vi "Read.vi"(8 "error in (no error)":errorcluster, 10 "maximum time (5s)":dbl[unit]=5000.0 caption="maximum time (5000 ms)", 11 "IVI_DMM in":refnum<class "IVI_DMM.lvclass">) -> (0 "error out":errorcluster, 2 "reading":dbl format="%^.2e", 3 "IVI_DMM out":refnum<class "IVI_DMM.lvclass">)   [LabVIEW 2013, in "IVI_DMM.lvlib" / "IVI_DMM.lvclass"]
doc: "This VI initiates a measurement, waits until the DMM has returned to the Idle state, and returns the measured value.\n\nThis VI applies default values to properties that have not been set by the user under the following conditions:\n\n(1) If the user has not set the value of any property in the IviDmmMultiPoint extension group, the VI sets the IviDmm>>Multi-Point Acquisition>>Sample Count [MP] and IviDmm>>Multi-Point Acquisition>>Trigger Count [MP] properties to 1.\n\n(2) If the user has not set the value of the IviDmm>Measurement Operation Options>Auto Zero [AZ] property, the VI sets the value of this property to IVIDMM_VAL_AUTO_ZERO_OFF (0). \n\nNotes:\n\n(1) After this VI executes, the Reading parameter contains an actual reading or a value indicating that an over-range condition occurred.\n\n(2) If an over-range condition occurs, the Reading parameter contains an IEEE defined NaN (Not a Number) value and the VI returns the IVIDMM_WARN_OVER_RANGE (0x3ffA2001) warning code.\n\n(3) You can test the measurement value for an over-range condition by calling the IviDmm Is Over-Range VI.\n\n(4) This VI performs interchangeability checking when the IviDmm>>Inherent IVI Settings>>User Options>>Interchange Check property is set to TRUE. If the IviDmm>>Inherent IVI Settings>>User Options>>Spy property is set to TRUE, you use the NI Spy utility to view interchangeability warnings. You use the IviDmm Get Next Interchange Warning VI to retrieve interchangeability warnings when the IviDmm>>Inherent IVI Settings>>User Options>>Spy property is set to FALSE. For more information about interchangeability checking, refer to the help text for the IviDmm>>Inherent IVI Settings>>User Options>>Interchange Check property.\n\n(5) The class driver returns a simulated measurement when this VI is called and the IviDmm>>Inherent IVI Settings>>User Options>>Simulate property is set to TRUE and the IviDmm>>Inherent IVI Settings>>User Options>>Use Specific Simulation property is set to FALSE. For information on how to configure a simulated measurement, refer to the online help manual."
uses:
  IVI_DMM.lvclass
  IVI_DMM.lvclass/IVI_DMM.ctl
  Base/CS++DMM/CS++DMM.lvclass/CS++DMM.ctl
  Base/CS++DMM/CS++DMM.lvclass
  Base/CS++DMM/Write reading.vi
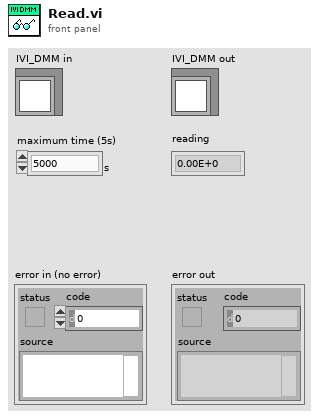
[diagram p1: front panel]
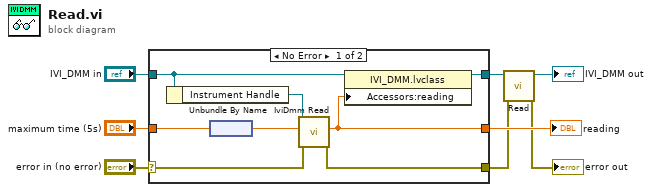
[diagram p0: block diagram]
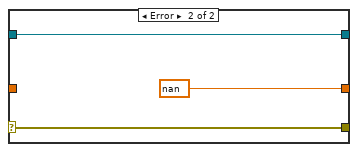
[diagram p2: hidden frame]
diagram:
  n1 = case shown="No Error" "error in (no error)" {
    selector: "error in (no error)" -> [w15 w19]
    tunnel: [w14 w19] -> w1
    tunnel: [w9 w18] -> w3
    tunnel: "IVI_DMM in" -> [w11 w18]
    tunnel: [w10 nan ("reading")] -> w6
    tunnel: "maximum time (5s)" -> [w13 _]
    frame No Error {
      n2 = Unbundle By Name(w11) -> ("Instrument Handle"=w16:refnum<k15>)
      n3 = node(w13) -> (w12:dbl)
      n4 = call <vilib>:"IviDmm Read.vi"("error in (no error)"=w15, "maximum time (5000 ms)"=w12, "instrument handle"=w16) -> ("error out"=w14:errorcluster, "reading"=w10:dbl)  [unwired: 6 in, 1 out]
      n5 = property class="IVI_DMM.lvclass"(reference=w11, "Accessors:reading"=w10) -> (reference out=w9:refnum<class "IVI_DMM.lvclass">)  [unwired: 1 in, 1 out]
    }
    frame Error {
    }
  }
  "reading" <- w6
  n6 = call-parent "Read.vi"("error in (no error)"=w1, "CS++DMM in"=w3) -> ("error out"=→"error out":errorcluster, "CS++DMM out"=→"IVI_DMM out":refnum<class "IVI_DMM.lvclass">)  [unwired: 7 in, 1 out]
